vi "ScaleSinewaveProp.vi"(1 "SineWave Properties":T2={"Sinewave Frequency (Hz)"=1000.0, "Phase Offset (deg)"=0.0, "Vpeak (V)"=10.0, "Voffset (V)"=0.0} {"Phase Offset (deg)" format="%#_6p"; "Sinewave Frequency (Hz)" format="%#_6p"}) -> (0 "Scaled Sinewave Props":T1)   [LabVIEW 2011]
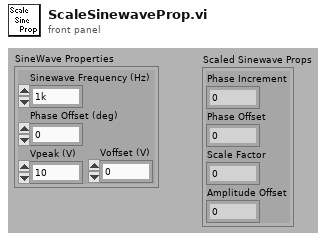
[diagram p1: front panel]
types:
  T1 = cluster{"Phase Increment":u32, "Phase Offset":u32, "Scale Factor":i16, "Amplitude Offset":i16}
  T2 = cluster{"Sinewave Frequency (Hz)":dbl, "Phase Offset (deg)":dbl, "Vpeak (V)":dbl, "Voffset (V)":dbl}
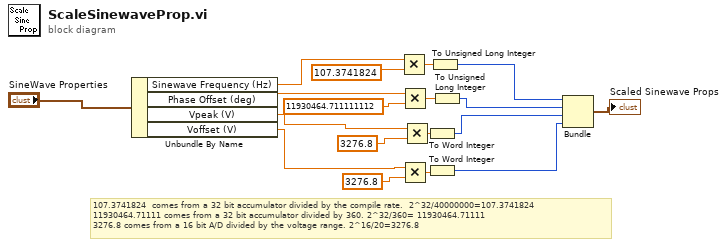
[diagram p0: block diagram]
diagram:
  # "107.3741824  comes from a 32 bit accumulator divided by the compile rate.  2^32/40000000=107.3741824\n11930464.71111 comes from a 32 bit accumulator divided by 360. 2^32/360= 11930464.71111\n3276.8 comes from a 16 bit A/D divided by the voltage range. 2^16/20=3276.8"
  n1 = Unbundle By Name("SineWave Properties") -> ("Sinewave Frequency (Hz)"=w15:dbl, "Phase Offset (deg)"=w16:dbl, "Vpeak (V)"=w17:dbl, "Voffset (V)"=w18:dbl)
  n2 = Multiply(x=w15, y=107.3741824) -> (x*y=w9:dbl)
  n3 = Multiply(x=w16, y=11930464.711111112) -> (x*y=w10:dbl)
  n4 = Multiply(x=w18, y=3276.8) -> (x*y=w7:dbl)
  n5 = Multiply(x=w17, y=3276.8) -> (x*y=w12:dbl)
  n6 = To Word Integer(number=w12) -> (16bit integer=w2:i16)
  n7 = To Word Integer(number=w7) -> (16bit integer=w1:i16)
  n8 = To Unsigned Long Integer(number=w9) -> (unsigned 32bit integer=w4:u32)
  n9 = To Unsigned Long Integer(number=w10) -> (unsigned 32bit integer=w3:u32)
  n10 = Bundle(w4, w3, w2, w1) -> (→"Scaled Sinewave Props":cluster{u32, u32, i16, i16})  [unwired: 1 out]
